vi "First_Program_2.vi"() -> ()   [LabVIEW 2012]
uses:
  Code/Control 1.ctl
  BotSpeakSubs/BotspeakSettingsUsed.vi
  <userlib>/BotSpeak/VIs/SubVIs/BotSpeak_Globals.vi
  SubVIs/LVPresent_Globals.vi
panel:
  in  "State":T1
  in  "Open":bool
  in  "Port":u8=13
  in  "Run":bool
  # "Writing LabVIEW Code\n\nPush the Run button - does the light built into the board turn on?  Change it from LO to HI - and run it again.  What happens? Try changing the Port - from pin 13 to pin 5. Note that the LO/HI states of the RGB LEDs is the opposite of the on-board LEDs. This is called a LabVIEW diagram - it is where your program resides - this program is simple - it changes the state of pin 13.  Once you open the program (click \"Open\") try clicking on the diagram, moving things around and see if you can break things."
  # "Click the open button to open the program and see more helpful tips!"
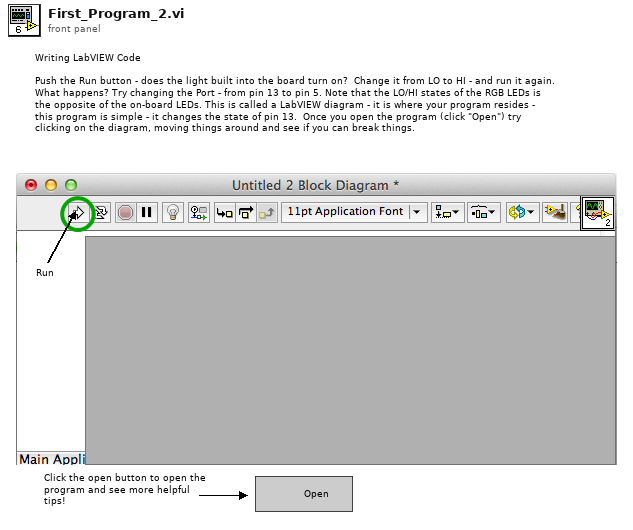
[diagram p1: front panel]
types:
  T1 = typedef "Control 1.ctl" = enum16{"LO", "HI"}
  T2 = typedef "BotSpeak_Control.ctl" = cluster{"Address":string, "Reply EOF":string, "Hardware":string, "Retries":i8, "Timeout":i32, "Open?":bool}
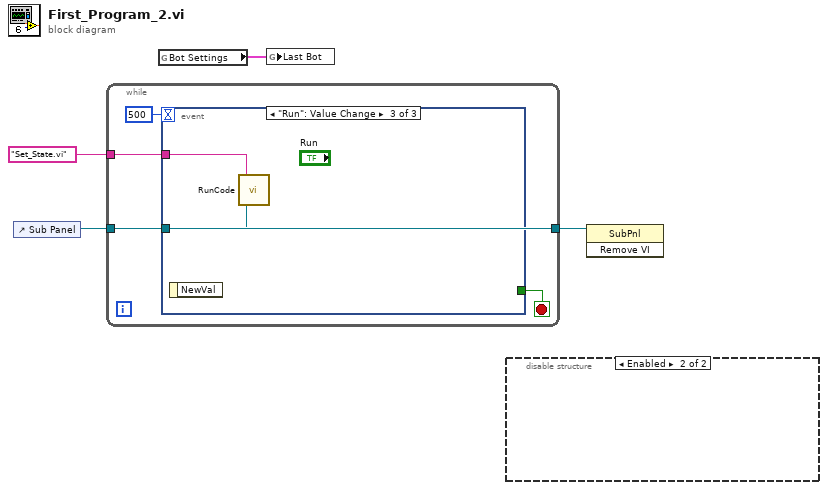
[diagram p0: block diagram]
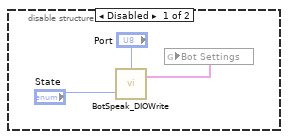
[diagram p2: hidden frame]
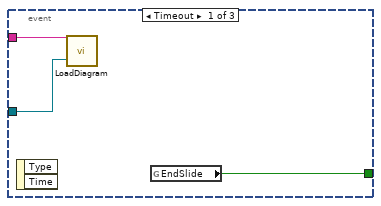
[diagram p3: hidden frame]
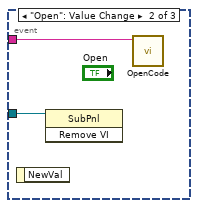
[diagram p4: hidden frame]
diagram:
  n1 = control-ref of="Sub Panel"() -> (w2:refnum<vi>)
  n2 = while {
    tunnel: "Set_State.vi" ("Code name") -> [w6]
    tunnel: w2 -> [w5]
    tunnel: [w5] -> w1
    stop <- w8 stop-if-true
    n3 = event shown="[2] \"Run\": Value Change" {
      selector: _ -> [_ _ _]
      dyn-events: _ -> [_ _ _]
      timeout: 500 -> [_ _ _]
      tunnel: [w11 _ _] -> w8
      tunnel: w6 -> [w9 w13 w15]
      tunnel: w5 -> [w10 w12 w14]
      event Timeout {
        n4 = event-data() -> ()  [unwired: 1 in, 2 out]
        n5 = call "LoadDiagram.vi"("SubPanel in"=w10, "Code name"=w9) -> ()  [unwired: 2 in]
        n6 = global read "LVPresent_Globals.vi" "EndSlide"() -> (w11:bool)
      }
      event "Open": Value Change {
        n7 = event-data() -> ()  [unwired: 1 in, 1 out]
        n8 = invoke class="SubPnl" method="Remove VI"(reference=w12) -> ()  [unwired: 2 in, 3 out]
        n9 = call "OpenCode.vi"("Code name"=w13) -> ()  [unwired: 3 in]
      }
      event "Run": Value Change {
        n10 = event-data() -> ()  [unwired: 1 in, 1 out]
        n11 = call "RunCode.vi"("SubPanel in"=w14, "Code name"=w15) -> ()  [unwired: 2 in]
      }
    }
  }
  n12 = global read "BotspeakSettingsUsed.vi" "Bot Settings"() -> (w4:T2)
  n13 = global write "BotSpeak_Globals.vi" "Last Bot"(w4) -> ()
  n14 = disable-structure shown="Enabled" {
    frame Disabled {
      n15 = call <userlib>:"BotSpeak_DIOWrite.vi"("State"="State", "DIO Line"="Port") -> (2:"Bot Settings"=w18:T2, 4:"Bot Settings"=w19:T2)  [unwired: 1 out]
      n16 = global write "BotspeakSettingsUsed.vi" "Bot Settings"(w19) -> ()
    }
    frame Enabled {
    }
  }
  n17 = invoke class="SubPnl" method="Remove VI"(reference=w1) -> ()  [unwired: 2 in, 3 out]
